vi "macro_HolDrvCtrl_New.vi"   [LabVIEW 2019, in "Trajectory_Library.lvlib"]
uses:
  Trajectory_Library.lvlib
types:
  T1 = typedef "Trajectory_Library.lvlib/PID_CONTROLLER.ctl" = cluster{"Kp":dbl, "Ki":dbl, "Kd":dbl, "Period":dbl, "Max_Integral":dbl, "Min_Integral":dbl, "Max_Input":dbl, "Min_Input":dbl, "Continuous":bool, "PositionError":dbl, "VelocityError":dbl, "PrevError":dbl, "TotalError":dbl, "PositionTolerance":dbl, "VelocityTolerance":dbl, "SetPoint":dbl, "Kf":dbl, "Prev_Deriv":dbl, "Prev_Deriv 2":dbl, "DerivativeFilter":bool, "Min_Output":dbl, "Max_Output":dbl, "Prev_F_P":dbl, "Prev_F_P_2":dbl, "AntiWindupActive":bool, "Measurement":dbl}
  T2 = typedef "Trajectory_Library.lvlib/TRAPEZOID_PROFILE_CONSTRAINT.ctl" = cluster{"MaxVelocity":dbl, "MaxAcceleration":dbl}
  T3 = typedef "Trajectory_Library.lvlib/PROFILED_PID_CONTROLLER.ctl" = cluster{"Controller":T1, "Goal":T4, "Setpoint":T4, "Constraint":T2}
  T4 = typedef "Trajectory_Library.lvlib/TRAPEZOID_PROFILE_STATE.ctl" = cluster{"Position":dbl, "Velocity":dbl}
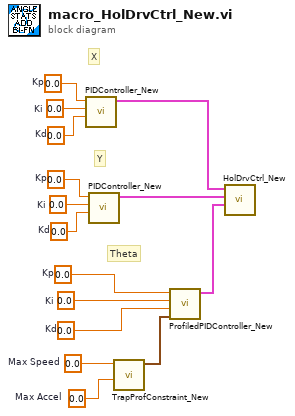
[diagram p0: block diagram]
diagram:
  w2 = 0.0  # Max Speed
  w3 = 0.0  # Max Accel
  w5 = 0.0  # Kp
  w6 = 0.0  # Ki
  w7 = 0.0  # Kd
  w10 = 0.0  # Kp
  w11 = 0.0  # Ki
  w12 = 0.0  # Kd
  w13 = 0.0  # Kp
  w14 = 0.0  # Ki
  w15 = 0.0  # Kd
  # "Theta"
  # "Y"
  # "X"
  n1 = call "PIDController_New.vi"("Kd"=w15, "Ki"=w14, "Kp"=w13) -> ("PID_CONTROLLER"=w9:T1)  [unwired: 8 in]
  n2 = call "PIDController_New.vi"("Kd"=w12, "Ki"=w11, "Kp"=w10) -> ("PID_CONTROLLER"=w8:T1)  [unwired: 8 in]
  n3 = call "TrapProfConstraint_New.vi"("Max Accel"=w3, "Max Speed (M/S)"=w2) -> ("TRAPEZOID_PROFILE_CONSTRAINT"=w4:T2)  [unwired: 9 in]
  n4 = call "ProfiledPIDController_New.vi"("Constraints"=w4, "Kd"=w7, "Ki"=w6, "Kp"=w5) -> ("PROFILED_PID_CONTROLLER"=w1:T3)  [unwired: 7 in]
  n5 = call "HolDrvCtrl_New.vi"("thetaProfiledPID_CTRL"=w1, "yPID_CTRL"=w8, "xPID_CTRL"=w9) -> ()  [unwired: 8 in, 1 out]
